vi "Serialize Tagged LLP Packet Data.vi"(0 "tagged llp packet":T1, 1 "reset":bool, 9 "input valid":bool, 12 "ready for output":bool) -> (4 "serialized data":u8[](array[numeric]), 6 "valid bytes":fxp<+,4,4>, 8 "end of packet":bool, 10 "output valid":bool, 14 "ready for input":bool)   [LabVIEW 2020, in "GettingStarted_Acq_Tap_148X_FPGA.lvlib"]
uses:
  GettingStarted_Acq_Tap_148X_FPGA.lvlib
  <instrlib>/FlexRIO/CSI-2/v2/FPGA/Types/Tagged LLP Packet.ctl
  <instrlib>/FlexRIO/CSI-2/v2/FPGA/Types/FPGA LLP Packet Tag.ctl
  <instrlib>/FlexRIO/CSI-2/v2/FPGA/Types/FPGA LLP Packet Timestamp.ctl
  <instrlib>/FlexRIO/CSI-2/v2/FPGA/Types/Timestamp ID.ctl
  <instrlib>/FlexRIO/CSI-2/v2/FPGA/Types/FPGA LLP Packet Size.ctl
  <instrlib>/FlexRIO/CSI-2/v2/FPGA/Types/LLP Packet.ctl
  <instrlib>/FlexRIO/CSI-2/v2/FPGA/Types/LLP Packet Header.ctl
  <instrlib>/FlexRIO/CSI-2/v2/FPGA/Types/LLP Packet Payload.ctl
  <instrlib>/FlexRIO/CSI-2/v2/FPGA/Types/LLP Packet Footer.ctl
  <instrlib>/FlexRIO/CSI-2/v2/FPGA/Types/Serialize Tagged LLP Packet State Data.ctl
  <instrlib>/FlexRIO/CSI-2/v2/FPGA/Types/Serialize Tagged LLP Packet State.ctl
  eec220a6-c820-4681-abd2-96deb8ceadbc.vi
  <instrlib>/FlexRIO/CSI-2/v2/FPGA/NI CSI-2 API FPGA v2.lvlib
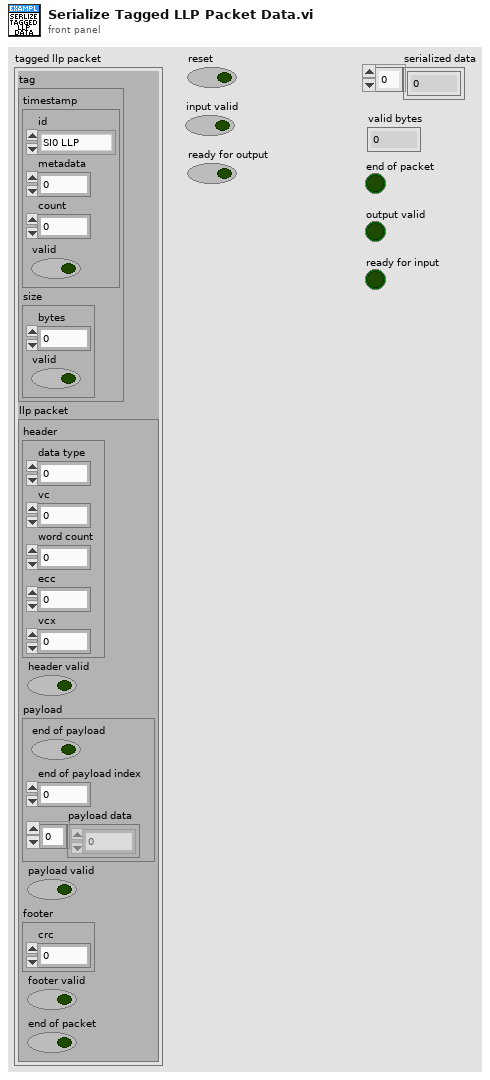
[diagram p1: front panel]
types:
  T1 = typedef "NI CSI-2 API FPGA v2.lvlib/Tagged LLP Packet.ctl" = cluster{"tag":T2, "llp packet":T6}
  T2 = typedef "NI CSI-2 API FPGA v2.lvlib/FPGA LLP Packet Tag.ctl" = cluster{"timestamp":T3, "size":T5}
  T3 = typedef "NI CSI-2 API FPGA v2.lvlib/FPGA LLP Packet Timestamp.ctl" = cluster{"valid":bool, "count":fxp<+,50,50>, "id":T4, "metadata":u8}
  T4 = typedef "NI CSI-2 API FPGA v2.lvlib/Timestamp ID.ctl" = enum8{"SI0 LLP", "SI1 LLP", "SI2 LLP", "SI3 LLP", "SI4 LLP", "SI5 LLP", "SI6 LLP", "SI7 LLP", "SO0 LLP", "SO1 LLP", "SO2 LLP", "SO3 LLP", "SO4 LLP", "SO5 LLP", "SO6 LLP", "SO7 LLP", "Ser0 GPIO Bank", "Ser1 GPIO Bank", "Ser2 GPIO Bank", "Ser3 GPIO Bank", "Ser4 GPIO Bank", "Ser5 GPIO Bank", "Ser6 GPIO Bank", "Ser7 GPIO Bank", "Des0 GPIO Bank", "Des1 GPIO Bank", "Des2 GPIO Bank", "Des3 GPIO Bank", "Des4 GPIO Bank", "Des5 GPIO Bank", "Des6 GPIO Bank", "Des7 GPIO Bank", "User0", "User1", "User2", "User3", "User4", "User5", "User6", "User7", "User8", "User9", "User10", "User11", "User12", "User13", "User14", "User15", "User16", "User17", "User18", "User19", "User20", "User21", "User22", "User23", "User24", "User25", "User26", "User27", "User28", "User29", "User30", "User31"}
  T5 = typedef "NI CSI-2 API FPGA v2.lvlib/FPGA LLP Packet Size.ctl" = cluster{"bytes":fxp<+,17,17>, "valid":bool}
  T6 = typedef "NI CSI-2 API FPGA v2.lvlib/LLP Packet.ctl" = cluster{"header":T7, "header valid":bool, "payload":T8, "payload valid":bool, "footer":T9, "footer valid":bool, "end of packet":bool}
  T7 = typedef "NI CSI-2 API FPGA v2.lvlib/LLP Packet Header.ctl" = cluster{"word count":u16, "ecc":fxp<+,6,6>, "vcx":fxp<+,2,2>, "data type":fxp<+,6,6>, "vc":fxp<+,2,2>}
  T8 = typedef "NI CSI-2 API FPGA v2.lvlib/LLP Packet Payload.ctl" = cluster{"end of payload":bool, "end of payload index":fxp<+,3,3>, "payload data":u8[]}
  T9 = typedef "NI CSI-2 API FPGA v2.lvlib/LLP Packet Footer.ctl" = cluster{"crc":u16}
  T10 = cluster{"serialized packet word":u8[], "valid bytes":fxp<+,4,4>, "end of packet":bool}
  T11 = typedef "NI CSI-2 API FPGA v2.lvlib/Serialize Tagged LLP Packet State.ctl" = enum8{"wait for header", "wait for end of packet"}
  T12 = typedef "NI CSI-2 API FPGA v2.lvlib/Serialize Tagged LLP Packet State Data.ctl" = cluster{"cache":u8[], "cache size":fxp<+,5,5>, "state":T11, "end of packet":bool}
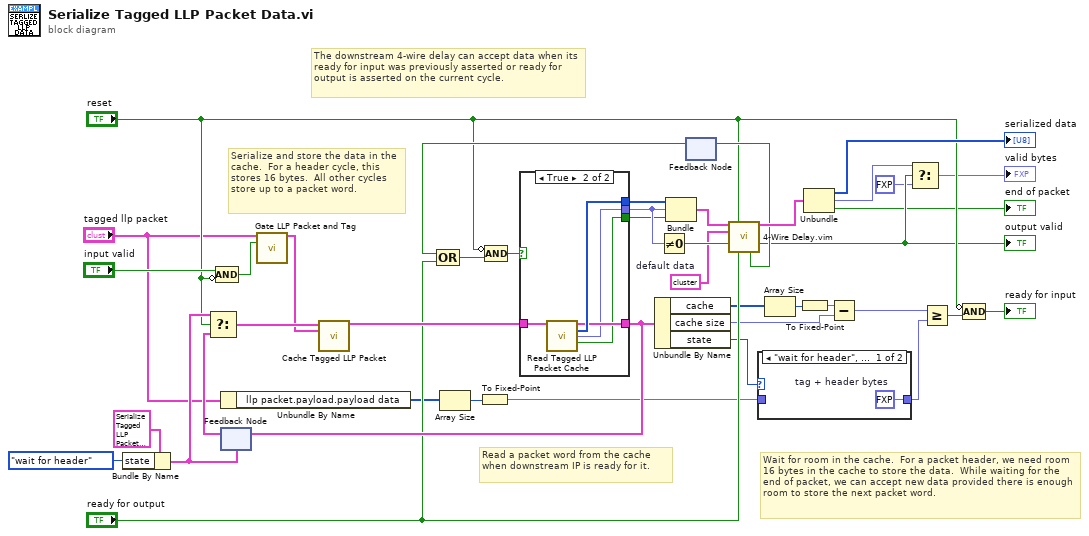
[diagram p0: block diagram]
diagram:
  w1 = T10 {"serialized packet word"=[0, 0, 0, 0, 0, 0, 0, 0], "valid bytes"=0.0, "end of packet"=FALSE}  # default data
  # "Serialize and store the data in the cache.  For a header cycle, this stores 16 bytes.  All other cycles store up to a packet word."
  # "Read a packet word from the cache when downstream IP is ready for it."
  # "Wait for room in the cache.  For a packet header, we need room 16 bytes in the cache to store the data.  While waiting for the end of packet, we can accept new data provided there is enough room to store the next packet word."
  # "The downstream 4-wire delay can accept data when its ready for input was previously asserted or ready for output is asserted on the current cycle."
  n1 = Bundle By Name(cluster=T12 {"cache"=[0, 0, 0, 0, 0, 0, 0, 0, 0, 0, 0, 0, 0, 0, 0, 0], "cache size"=0.0, "state"=enum."wait for header", "end of packet"=FALSE}, "state"=Serialize_Tagged_LLP_Packet_State."wait for header") -> (w37:T12)
  n2 = Compound Arithmetic op=AND("input valid", invert "reset") -> (w40:bool)
  n3 = Unbundle By Name("tagged llp packet") -> ("llp packet.payload.payload data"=w6:u8[])
  n4 = feedback #1(w37) -> (w36:T12)
  n5 = Select(t=w37, s="reset", f=w36) -> (s? t:f=w26:T12)
  n6 = call <instrlib>:"Gate LLP Packet and Tag.vi"("tagged llp packet in"="tagged llp packet", "enable"=w40) -> ("tagged llp packet out"=w5:T1)  [unwired: 13 in]
  n7 = call "Cache Tagged LLP Packet.vi"("state in"=w26, "tag llp packet"=w5) -> ("state out"=w42:T12)  [unwired: 13 in]
  n8 = Array Size(array=w6) -> (size(s)=w4:i32)
  n9 = To Fixed-Point(number=w4) -> (fixed-point=w3:fxp<+,5,5>)  [unwired: 1 in]
  n10 = feedback #2() -> (w28:bool)  [unwired: 1 in]
  n11 = Compound Arithmetic op=OR(w28, "ready for output") -> (w33:bool)
  n12 = Compound Arithmetic op=AND(invert "reset", w33) -> (w34:bool)
  n13 = case shown="True" w34 {
    tunnel: w42 -> [w43 w45]
    tunnel: [_ w48] -> w25
    tunnel: [_ w46] -> w24
    tunnel: [w43 w47] -> w35
    tunnel: [_ w44] -> w8
    frame False {
    }
    frame True {
      n14 = call "Read Tagged LLP Packet Cache.vi"("state in"=w45) -> ("state out"=w47:T12, "serialized packet word"=w48:u8[], "valid bytes"=w46:fxp<+,4,4>, "end of packet"=w44:bool)  [unwired: 11 in]
    }
  }
  n15 = feedback-in #1(w35) -> ()
  n16 = Unbundle By Name(w35) -> ("cache"=w18:u8[], "cache size"=w17:fxp<+,5,5>, "state"=w14:T11)
  n17 = Not Equal To 0?(x=w24) -> (x != 0?=w32:bool)
  n18 = Bundle("serialized packet word"=w25, "valid bytes"=w24, "end of packet"=w8) -> (w31:T10)  [unwired: 1 in]
  n19 = call "4-Wire Delay.vim"("data in"=w31, "reset"="reset", "default data"=w1, "input valid"=w32, "ready for output"="ready for output") -> ("data out"=w30:T10, "output valid"=w10:bool, "ready for input"=w29:bool)  [unwired: 8 in]
  "output valid" <- w10
  n20 = feedback-in #2(w29) -> ()
  n21 = case shown="\"wait for header\", Default" w14 {
    tunnel: [w49 w50] -> w13
    tunnel: w3 -> [_ w50]
    frame "wait for header", Default {
      w49 = fxp<+,5,5> 16.0  # tag + header bytes
    }
    frame "wait for end of packet" {
    }
  }
  n22 = Array Size(array=w18) -> (size(s)=w22:i32)
  n23 = To Fixed-Point(number=w22) -> (fixed-point=w21:fxp<+,5,5>)  [unwired: 1 in]
  n24 = Unbundle(w30) -> ("serialized packet word"=→"serialized data":u8[], "valid bytes"=w12:fxp<+,4,4>, "end of packet"=→"end of packet":bool)
  n25 = Subtract(x=w21, y=w17) -> (x-y=w20:fxp<+,5,5>)
  n26 = Select(t=w12, s=w10, f=fxp<+,4,4> 0.0) -> (s? t:f=→"valid bytes":fxp<+,4,4>)
  n27 = Greater Or Equal?(x=w20, y=w13) -> (x >= y?=w19:bool)
  n28 = Compound Arithmetic op=AND(invert "reset", w19) -> (→"ready for input":bool)
